vi "failUnless.vi"(8 "error in (no error)":errorcluster, 9 "message (\"\")":string, 10 "pass":bool, 11 "TestCase in":refnum<class "TestCase.lvclass">) -> (0 "error out":errorcluster, 3 "TestCase out":refnum<class "TestCase.lvclass">)   [LabVIEW 2013, in "TestCase.lvclass"]
doc: "{Obsolete - kept for compatiblity only}\n\nFail if 'pass' condition is FALSE. On failure, 'message' is appended to failure status."
uses:
  TestCase.lvclass
panel:
  # "JKI VI Tester for LabVIEW\nhttp://jkisoft.com/vi-tester\nCopyright (C) 2007-2009, JKI <info@jkisoft.com>\nALL RIGHTS RESERVED"
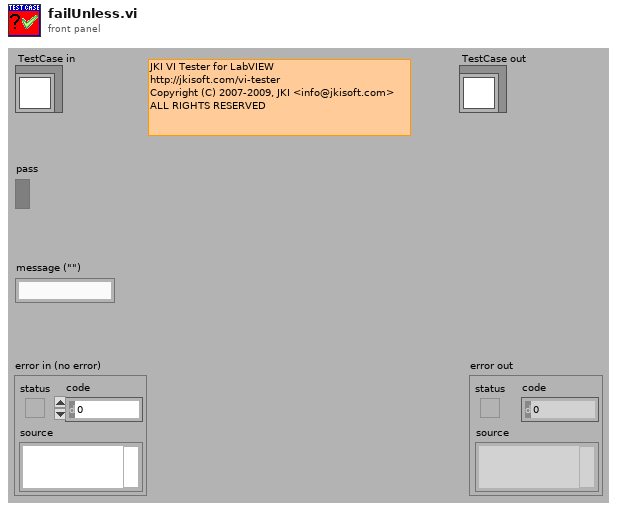
[diagram p1: front panel]
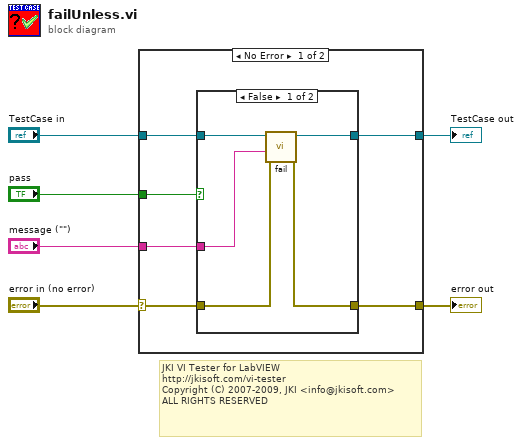
[diagram p0: block diagram]
diagram:
  # "JKI VI Tester for LabVIEW\nhttp://jkisoft.com/vi-tester\nCopyright (C) 2007-2009, JKI <info@jkisoft.com>\nALL RIGHTS RESERVED"
  n1 = case shown="No Error" "error in (no error)" {
    selector: "error in (no error)" -> [w12 w21]
    tunnel: [w11 w21] -> w2
    tunnel: [w7 w20] -> w3
    tunnel: "TestCase in" -> [w8 w20]
    tunnel: "message (\"\")" -> [w10 _]
    tunnel: "pass" -> [w9 _]
    frame No Error {
      n2 = case shown="False" w9 {
        tunnel: w12 -> [w17 w19]
        tunnel: [w16 w19] -> w11
        tunnel: w10 -> [w15 _]
        tunnel: w8 -> [w14 w18]
        tunnel: [w13 w18] -> w7
        frame False {
          n3 = call-dynamic "fail.vi"("error in (no error)"=w17, "message (\"\")"=w15, "TestCase in"=w14) -> ("error out"=w16:errorcluster, "TestCase out"=w13:refnum<class "TestCase.lvclass">)  [unwired: 7 in]
        }
        frame True {
        }
      }
    }
    frame Error {
    }
  }
  "error out" <- w2
  "TestCase out" <- w3
